vi "Read Digio Bit_mx.vi"(7 "error in":errorcluster, 8 "line":i16, 10 "DI Task":refnum<k21>) -> (0 "error out":errorcluster, 3 "line state":bool)   [LabVIEW 2010]
uses:
  <vilib>/DAQmx/read.llb/DAQmx Read (Digital 1D Bool NChan 1Samp 1Line).vi
  <vilib>/daqmx/miscellaneous.llb/DAQmx Fill In Error Info.vi
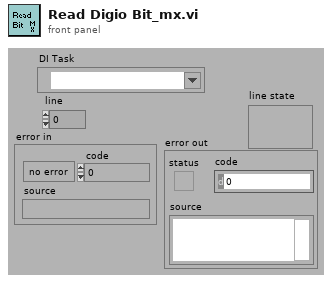
[diagram p1: front panel]
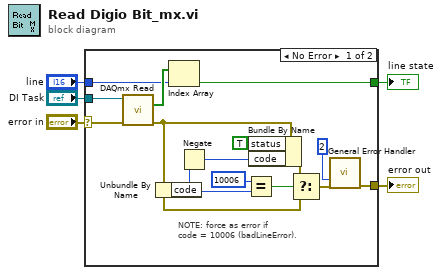
[diagram p0: block diagram]
diagram:
  n1 = case shown="No Error" "error in" {
    selector: "error in" -> [w10 w21]
    tunnel: "DI Task" -> [w12 _]
    tunnel: "line" -> [w7 _]
    tunnel: [w9 w21] -> w1
    tunnel: [w6 _] -> w2
    frame No Error {
      # "NOTE: force as error if\ncode = 10006 (badLineError)."
      n2 = call-poly <vilib>:"DAQmx Read.vi"("task/channels in"=w12, "error in"=w10) -> ("data"=w8:bool[], "error out"=w11:errorcluster)  [unwired: 11 in, 1 out]
      n3 = Unbundle By Name(w11) -> ("code"=w15:i32)
      n4 = Index Array(array=w8, index=w7) -> (element=w6:bool)
      n5 = Negate(x=w15) -> (-x=w17:i32)
      n6 = Equal?(x=10006, y=w15) -> (x = y?=w19:bool)
      n7 = Bundle By Name(cluster=w11, "status"=TRUE, "code"=w17) -> (w14:errorcluster)
      n8 = Select(t=w14, s=w19, f=w11) -> (s? t:f=w16:errorcluster)
      n9 = call <vilib>:"General Error Handler.vi"("type of dialog (OK msg:1)"=u16 2, "error in (no error)"=w16) -> ("error out"=w9:errorcluster)  [unwired: 9 in, 4 out]
    }
    frame Error {
    }
  }
  "line state" <- w2
  "error out" <- w1
